vi "test 64 Bit 20xx Version.vi"(8 "error in (no error)":errorcluster, 11 "TestCase in":refnum<class "Get LabVIEW Version Tests.lvclass">) -> (0 "error out":errorcluster, 3 "TestCase out":refnum<class "Get LabVIEW Version Tests.lvclass">)   [LabVIEW 2015, in "Get LabVIEW Version Tests.lvclass"]
uses:
  Get LabVIEW Version Tests.lvclass
  <vilib>/addons/_JKI Toolkits/VI Tester/TestCase.llb/TestCase.lvclass
  G CLI VIP.lvlib
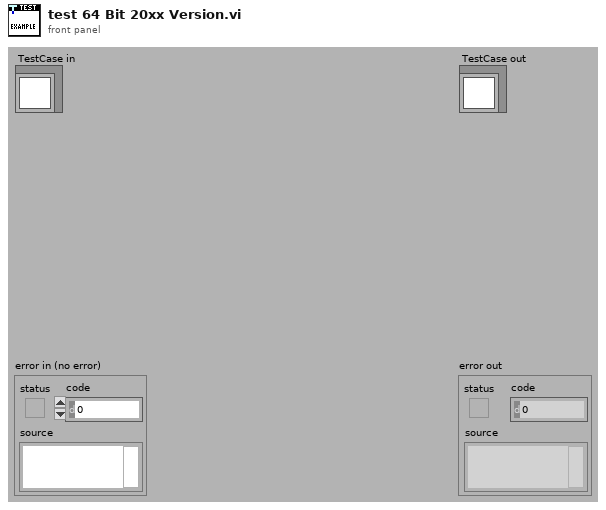
[diagram p1: front panel]
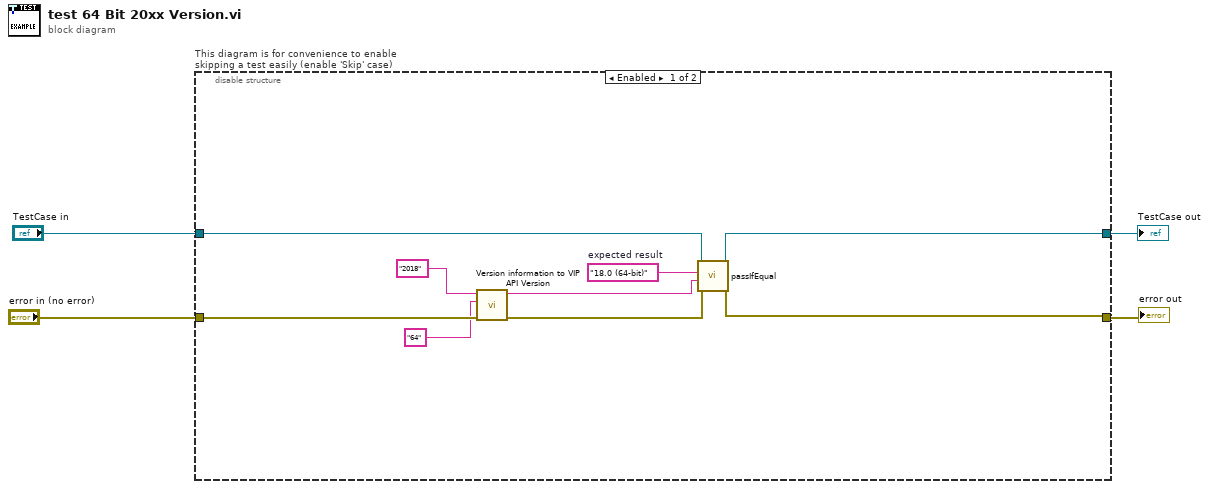
[diagram p0: block diagram]
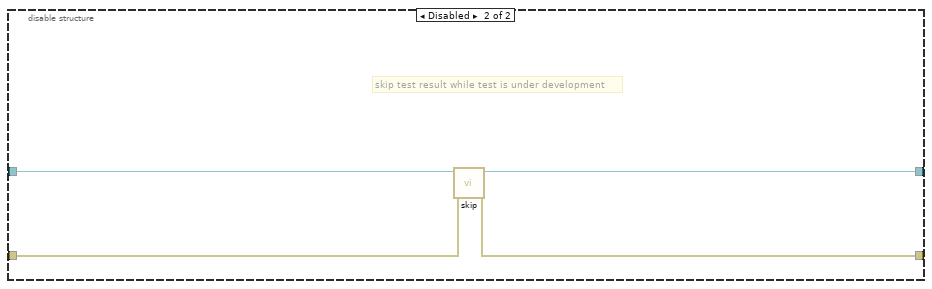
[diagram p2: hidden frame]
diagram:
  n1 = disable-structure "This diagram is for convenience to enable skipping a test easily (enable 'Skip' case)" shown="Enabled" {
    disable-tunnel: "TestCase in" -> [w12 w17]
    disable-tunnel: [w11 w15] -> w1
    disable-tunnel: [w10 w16] -> w3
    disable-tunnel: "error in (no error)" -> [w9 w14]
    frame Enabled {
      w13 = "18.0 (64-bit)"  # expected result
      n2 = call "Version information to VIP API Version.vi"("error in (no error)"=w9, "Bitness String"="64" ("Version String"), "Version String"="2018") -> ("error out"=w8:errorcluster, "VIP Version"=w7:string)  [unwired: 7 in]
      n3 = call-dynamic "passIfEqual.vi"("error in (no error)"=w8, "y"=w7, "x"=w13, "TestCase in"=w12) -> ("error out"=w10:errorcluster, "TestCase out"=w11:refnum<class "Get LabVIEW Version Tests.lvclass">)  [unwired: 6 in]
    }
    frame Disabled {
      # "skip test result while test is under development"
      n4 = call <vilib>:"skip.vi"("error in (no error)"=w14, "TestCase in"=w17) -> ("error out"=w16:errorcluster, "TestCase out"=w15:refnum<class "Get LabVIEW Version Tests.lvclass">)  [unwired: 8 in]
    }
  }
  "error out" <- w3
  "TestCase out" <- w1
